vi "get.FieldSpec.by.Name.vi"(8 "error in (no error)":errorcluster, 10 "Field.Name":string="Length", 11 "PitchMessage in":refnum<class "PitchMessage.lvclass">) -> (0 "error out":errorcluster, 2 "Index":i32, 3 "PitchMessage out":refnum<class "PitchMessage.lvclass">)   [LabVIEW 2020, in "PitchMessage.lvclass"]
uses:
  PitchMessage.lvclass
  PitchMessage.lvclass/PitchMessage.ctl
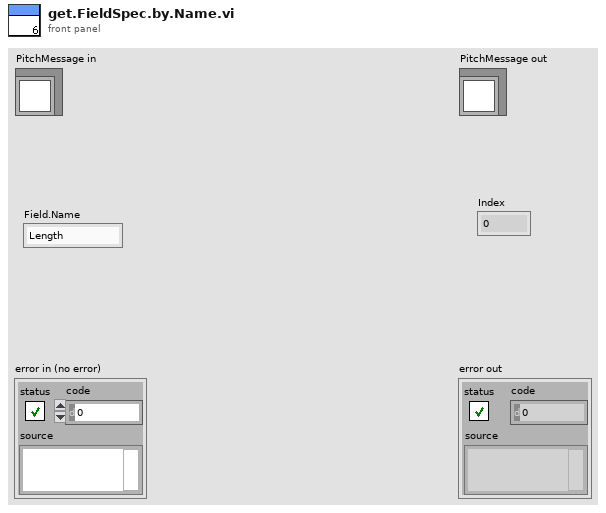
[diagram p1: front panel]
types:
  T1 = typedef "FieldSpec.ctl" = cluster{"Name":string, "Offset":i32, "Length":i32, "FieldType":enum16{"Alphanumeric", "Binary", "BinaryLongPrice", "BinaryShortPrice", "BitField", "PrintableAscii", "Value"}, "FieldValue":variant}
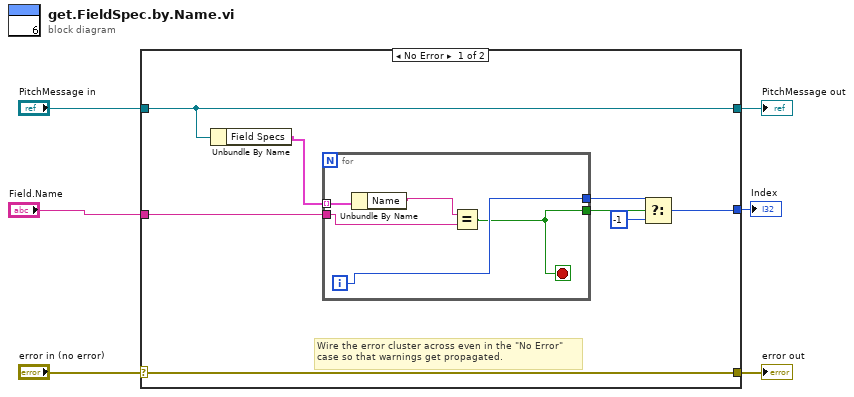
[diagram p0: block diagram]
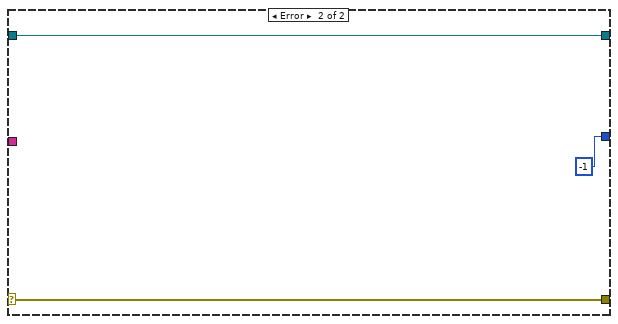
[diagram p2: hidden frame]
diagram:
  n1 = case shown="No Error" "error in (no error)" {
    selector: "error in (no error)" -> [w14 w22]
    tunnel: [w14 w22] -> w5
    tunnel: [w13 w21] -> w3
    tunnel: "PitchMessage in" -> [w13 w21]
    tunnel: [w8 -1] -> w2
    tunnel: "Field.Name" -> [w11 _]
    frame No Error {
      # "Wire the error cluster across even in the \"No Error\"\ncase so that warnings get propagated."
      n2 = Unbundle By Name(w13) -> ("Field Specs"=w12:T1[])
      n3 = for {
        tunnel: w12 -> [w19] mode=indexing
        tunnel: [w17] -> w9
        tunnel: w11 -> [w16]
        tunnel: [w15] -> w10
        i -> [w17]
        stop <- w15 stop-if-true
        n4 = Unbundle By Name(w19) -> ("Name"=w18:string)
        n5 = Equal?(x=w18, y=w16) -> (x = y?=w15:bool)
      }
      n6 = Select(t=w9, s=w10, f=-1) -> (s? t:f=w8:i32)
    }
    frame Error {
    }
  }
  "error out" <- w5
  "PitchMessage out" <- w3
  "Index" <- w2
